vi "Read Channel List.vi"(8 "error in":errorcluster, 11 "CIFChannelMng in":refnum<class "CIFChannelMng.lvclass">) -> (0 "error out":errorcluster, 2 "Channel List":T1[](array[typedef]) {"Custom Config Data" format="%.0x"}, 3 "CIFChannelMng out":refnum<class "CIFChannelMng.lvclass">)   [LabVIEW 2021, in "CIFChannelMng.lvclass"]
uses:
  CIFChannelMng.lvclass
  CIFChannelMng.lvclass/CIFChannelMng.ctl
  <vilib>/CIF Foundation/CIF Channels Core/ChannelCommon/typedef/Direction.ctl
  <vilib>/CIF Foundation/CIF Channels Core/ChannelCommon/ChannelCommon.lvlib
  typedef/Channel List for OOB.ctl
  <vilib>/CIF Foundation/CIF Channels Core/ChannelCommon/typedef/Channel Pattern.ctl
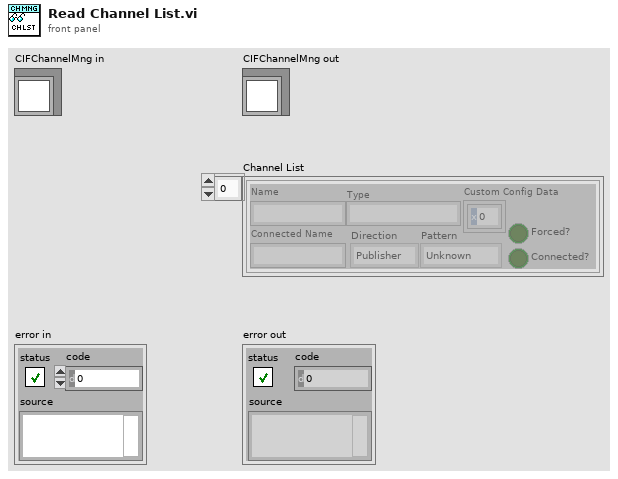
[diagram p1: front panel]
types:
  T1 = typedef "CIFChannelMng.lvclass/Channel List for OOB.ctl" = cluster{"Name":string, "Direction":T2, "Type":string, "Connected?":bool, "Connected Name":string, "Custom Config Data":u8[], "Forced?":bool, "Pattern":T3}
  T2 = typedef "ChannelCommon.lvlib/Direction.ctl" = enum8{"Publisher", "Subscriber"}
  T3 = typedef "ChannelCommon.lvlib/Channel Pattern.ctl" = enum8{"Unknown", "Tag", "FIFO", "MultiFIFO", "BackpressureFIFO"}
  T4 = typedef "CIFChannelMng.lvclass/TX DVR Data.ctl" = cluster{"Channel List":T1[], "Publisher Instance":T5}
  T5 = typedef "CIFChannelMng.lvclass/FIFO Publisher Return.ctl" = cluster{"FIFO Instance Config":T6, "error":errorcluster, "Added":bool}
  T6 = typedef "ChannelCommon.lvlib/New FIFO Instance Response.ctl" = cluster{"Publisher":string, "Custom Data":u8[]}
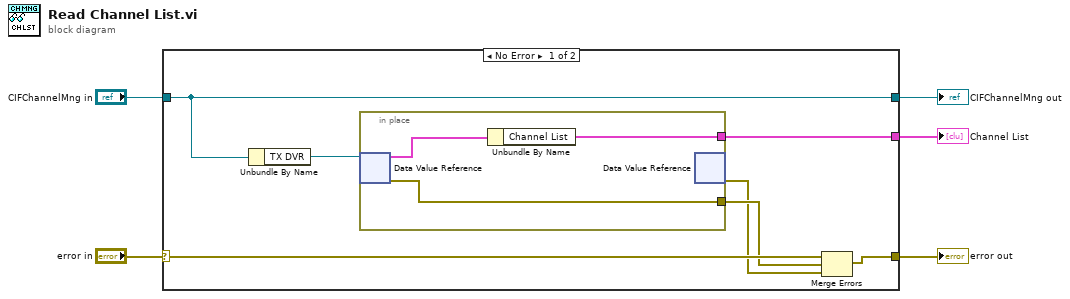
[diagram p0: block diagram]
diagram:
  n1 = case shown="No Error" "error in" {
    selector: "error in" -> [w10 w17]
    tunnel: [w6 w17] -> w3
    tunnel: "CIFChannelMng in" -> [w12 w16]
    tunnel: [w12 w16] -> w4
    tunnel: [w9 _] -> w1
    frame No Error {
      n2 = Unbundle By Name(w12) -> ("TX DVR"=w11:refnum<data-value>)
      n3 = in-place {
        in-place-border: [w14] -> w9
        in-place-border: [w13] -> w8
        n4 = in-place-dvr #1(w11) -> (w15:T4, w13:errorcluster)
        n5 = Unbundle By Name(w15) -> ("Channel List"=w14:T1[])
        n6 = in-place-dvr #1() -> (w7:errorcluster)  [unwired: 1 in, 1 out]
      }
      n7 = Merge Errors(w10, w8, w7) -> (w6:errorcluster)
    }
    frame Error {
    }
  }
  "error out" <- w3
  "Channel List" <- w1
  "CIFChannelMng out" <- w4
